vi "gfitsio-delete-hdu.vi"(4 "error in (no error)":errorcluster, 7 "gfits refnum":T1) -> (0 "error out":errorcluster, 1 "tbltype":i32(ring) items=["ASCII_TBL", "BINARY_TBL"], 3 "dup gfits refnum":T1)   [LabVIEW 2011, in "gfitsio.lvlib"]
doc: "Create a new bintable table extension. If the FITS file is currently empty then a dummy primary array will be created before appending the table extension to it. The initial number of rows is set equal to zero because CFITSIO will automatically increase the size of the table as additional rows are written. Any printable ASCII charaters may be used in the HDU name."
uses:
  gfitsio.lvlib
  gfitsio.dll
  Documents and Settings/ggatling/My Documents/p4depot/LabVIEW 8.5/applications/LP_ONESHOT/user.lib/gfitsio/gfitsio-refnum.ctl
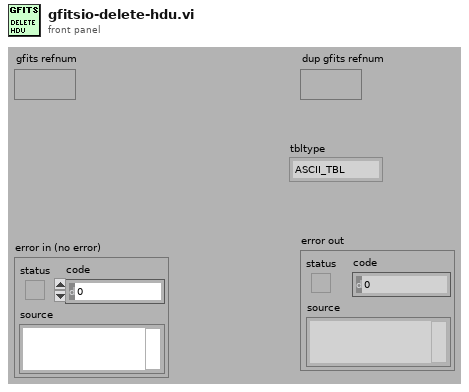
[diagram p1: front panel]
types:
  T1 = typedef "gfitsio-refnum.ctl" = refnum<k1>
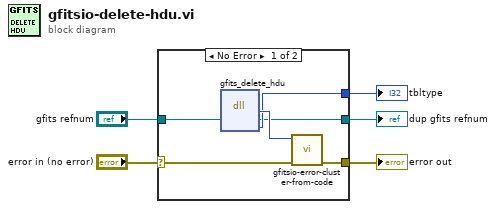
[diagram p0: block diagram]
diagram:
  n1 = case shown="No Error" "error in (no error)" {
    selector: "error in (no error)" -> [w9 w13]
    tunnel: [w11 w13] -> w5
    tunnel: "gfits refnum" -> [w6 w12]
    tunnel: [w7 w12] -> w3
    tunnel: [w8 _] -> w1
    frame No Error {
      n2 = dll-call lib="C:/BonOMM/SubVIs/gfitsio/gfitsio.dll" fn="gfits_delete_hdu"("gfits refnum"=w6) -> (w10:i32, "gfits refnum"=w7:T1, "tbltype"=w8:i32)  [unwired: 4 in, 2 out]
      n3 = call "gfitsio-error-cluster-from-code.vi"("error in (no error)"=w9, "error code"=w10) -> ("error out"=w11:errorcluster)  [unwired: 5 in]
    }
    frame Error {
    }
  }
  "error out" <- w5
  "dup gfits refnum" <- w3
  "tbltype" <- w1
